vi "(6) StepNLoop.vi"   [LabVIEW 2020]
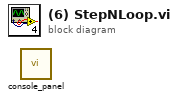
[diagram p0: block diagram]
diagram:
  n1 = call <instrlib>:"console_panel.vi"() -> ()  [unwired: 1 in]
